vi "BDR_Query.vi"(0 "System no.":i32=1 min=1 step=1, 5 "error in":errorcluster) -> (14 "Baudrate":dbl format="%.3f", 19 "error out":errorcluster)   [LabVIEW 2020]
doc: "Returns current RAM baud rate setting for RS-232 communication. \n\nE-755: The value returned reflects the value that is currently in effect. This value will be saved to non-volatile memory if parameters are saved with WPA.vi. Returned baud rate value is baud.\n\nE-816: The value returned reflects the value that will be saved to non-volatile memory if parameters are saved with WPA.vi. This may differ from the value currently in effect. Returned Baudrate value is in kbaud.\nThis command cannot be issued to a slave."
panel:
  # "Returns current RAM baudrate setting for RS-232 communication."
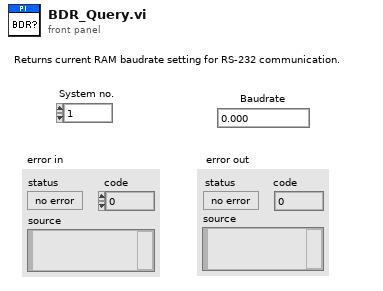
[diagram p1: front panel]
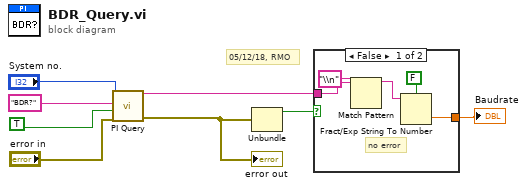
[diagram p0: block diagram]
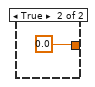
[diagram p2: hidden frame]
diagram:
  # "05/12/18, RMO"
  n1 = call "PI Query.vi"("System no."="System no.", "String to send"="BDR?", "Attach termination char.?"=TRUE ("Attach Linefeed?"), "error in"="error in") -> ("String read"=w2:string, "error out"=w1:errorcluster)  [unwired: 3 in, 11 out]
  "error out" <- w1
  n2 = Unbundle(w1) -> ("status"=w7:bool)  [unwired: 2 out]
  n3 = case shown="False" w7 {
    tunnel: w2 -> [w13 _]
    tunnel: [w9 0.0] -> w6
    frame False {
      # "no error"
      n4 = Match Pattern(string=w13, regular expression="\\n") -> (before substring=w10:string)  [unwired: 4 out]
      n5 = Fract/Exp String To Number(use system decimal point (T)=FALSE, string=w10) -> (number=w9:dbl)  [unwired: 3 out]
    }
    frame True {
    }
  }
  "Baudrate" <- w6
